vi "Parse Root.vi"(8 "error in (no error)":errorcluster, 11 "Alpaca CLI Parser in":refnum<class "JSON Parser.lvclass">) -> (0 "error out":errorcluster, 3 "Alpaca CLI Parser out":refnum<class "JSON Parser.lvclass">)   [LabVIEW 2019, in "JKI JSON Serialization.lvlib" / "JSON Parser.lvclass"]
doc: "JKI JSON 1.1.10.37\nTomi Maila - JKI\nCopyright (c) 2017, JKI"
uses:
  JSON Parser.lvclass
  JSON Parser.lvclass/JSON Parser.ctl
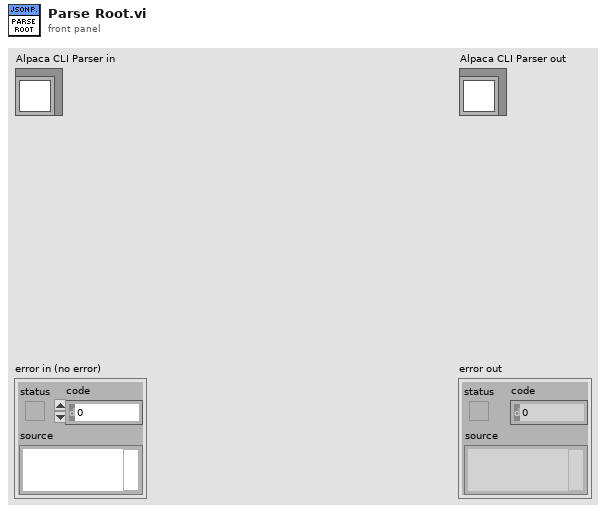
[diagram p1: front panel]
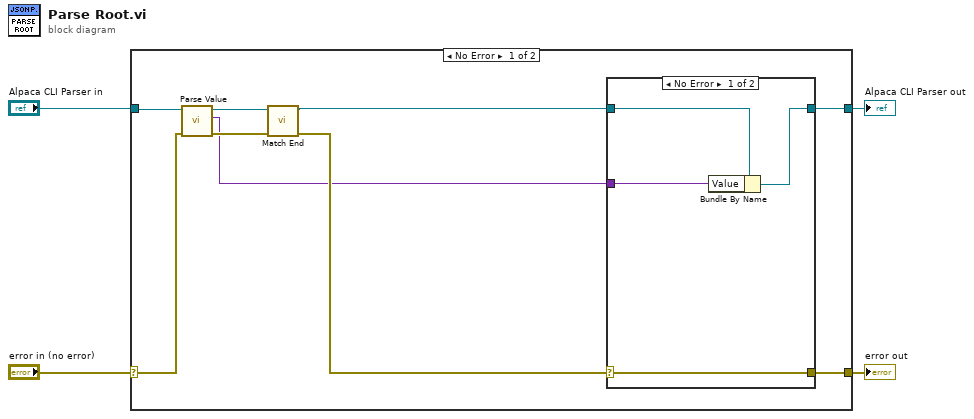
[diagram p0: block diagram]
diagram:
  n1 = case shown="No Error" "error in (no error)" {
    selector: "error in (no error)" -> [w11 w21]
    tunnel: [w8 w21] -> w3
    tunnel: [w13 w20] -> w1
    tunnel: "Alpaca CLI Parser in" -> [w12 w20]
    frame No Error {
      n2 = call-dynamic "Parse Value.vi"("error in (no error)"=w11, "Alpaca CLI Parser in"=w12) -> ("error out"=w9:errorcluster, "Value"=w5:variant, "Alpaca CLI Parser out"=w10:refnum<class "JSON Parser.lvclass">)  [unwired: 7 in]
      n3 = call-dynamic "Match End.vi"("error in (no error)"=w9, "Alpaca JSON Parser in"=w10) -> ("error out"=w6:errorcluster, "Alpaca JSON Parser out"=w7:refnum<class "JSON Parser.lvclass">)  [unwired: 8 in]
      n4 = case shown="No Error" w6 {
        selector: w6 -> [w15 w19]
        tunnel: [w17 w18] -> w13
        tunnel: [w15 w19] -> w8
        tunnel: w7 -> [w16 w18]
        tunnel: w5 -> [w14 _]
        frame No Error {
          n5 = Bundle By Name(cluster=w16, "Value"=w14) -> (w17:refnum<class "JSON Parser.lvclass">)
        }
        frame Error {
        }
      }
    }
    frame Error {
    }
  }
  "error out" <- w3
  "Alpaca CLI Parser out" <- w1
